vi "load system configuration.vi"(8 "error in":errorcluster) -> (0 "error out":errorcluster)   [LabVIEW 2015]
uses:
  global variables/params.vi
  <vilib>/Utility/config.llb/Read Key (String).vi
  <vilib>/Utility/config.llb/NI_LVConfig.lvlib
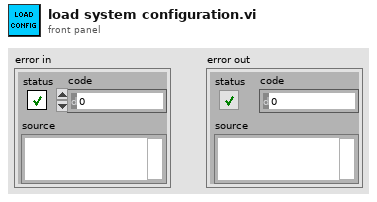
[diagram p1: front panel]
types:
  T1 = typedef "NI_LVConfig.lvlib/Config Data RefNum.ctl" = refnum<k1>
  T2 = cluster{"String":string, string, dbl, dbl, string, string, string, dbl, string}[]
  T3 = cluster{"String":string, string, dbl, dbl, string, string, string, dbl, string}
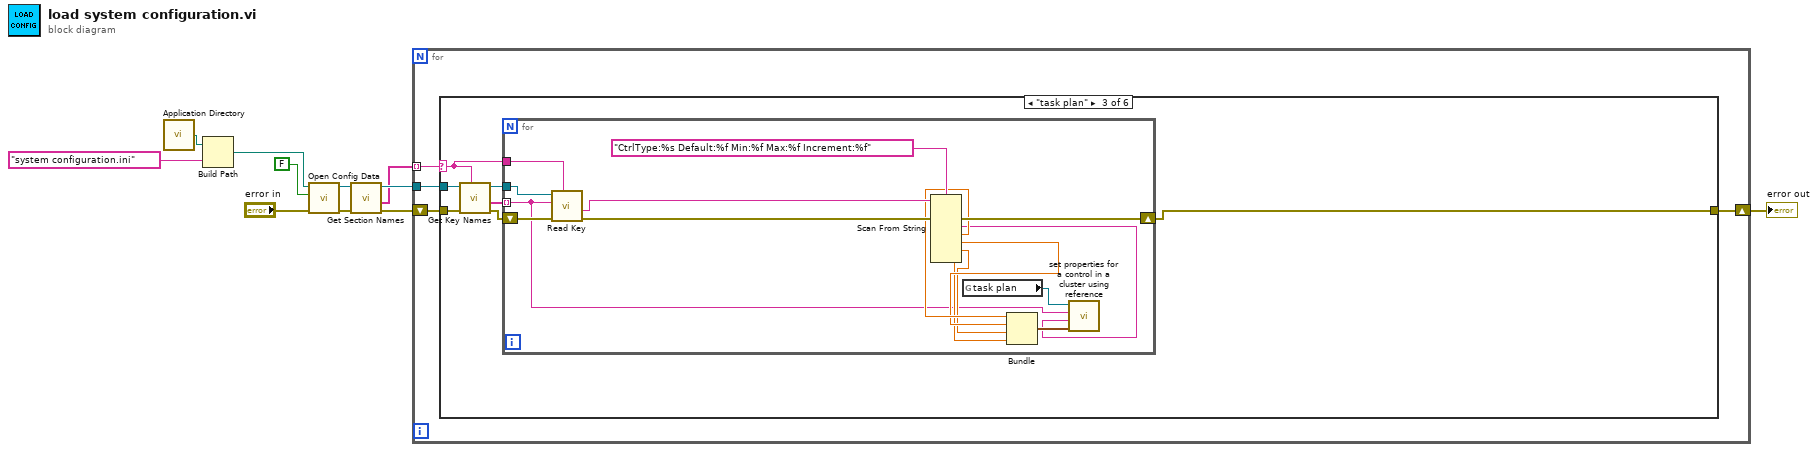
[diagram p0: block diagram]
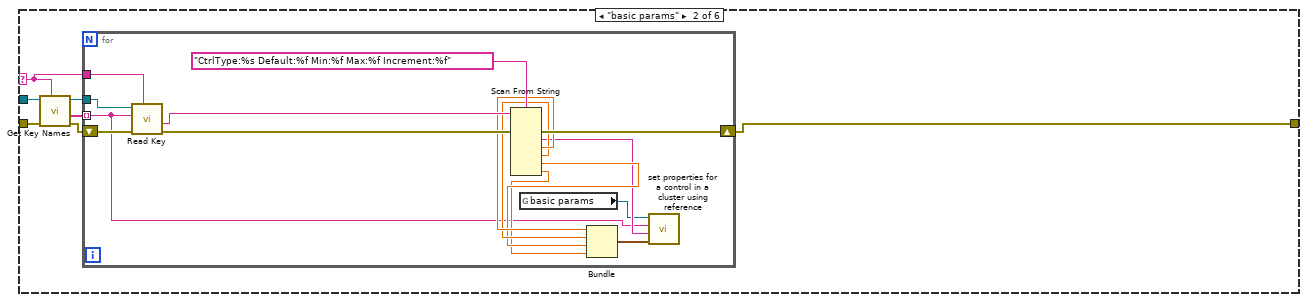
[diagram p3: hidden frame]
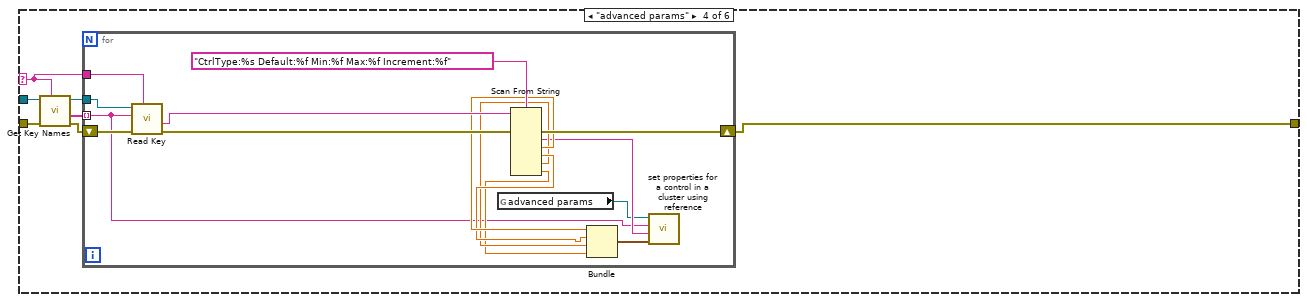
[diagram p4: hidden frame]
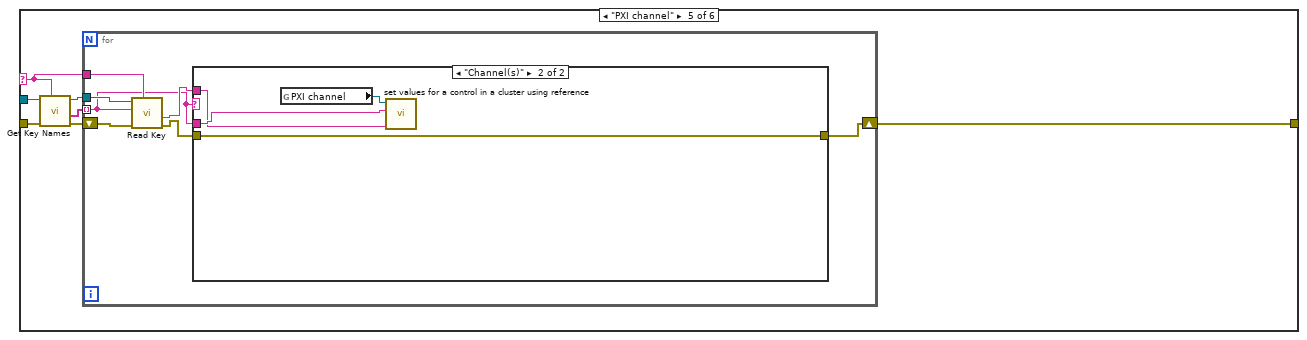
[diagram p5: hidden frame]
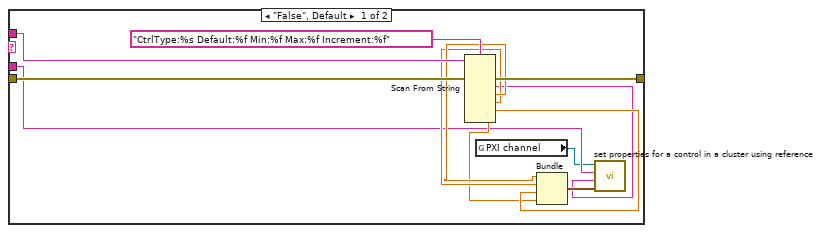
[diagram p6: hidden frame]
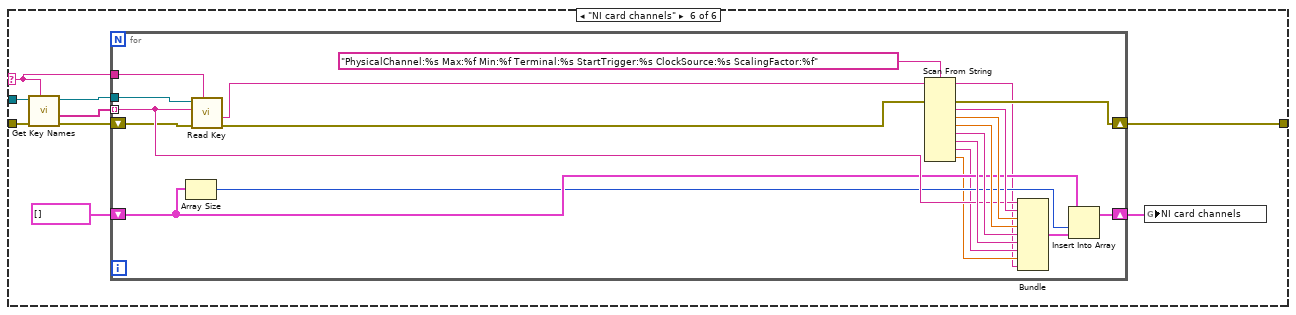
[diagram p7: hidden frame]
diagram:
  n1 = call <vilib>:"Application Directory.vi"() -> ("Application Directory"=w10:path)
  n2 = Build Path(base path=w10, name or relative path="system configuration.ini") -> (appended path=w8:path)
  n3 = call <vilib>:"Open Config Data.vi"("error in (no error)"="error in", "create file if necessary (T)"=FALSE, "configuration file path"=w8) -> ("error out"=w6:errorcluster, "refnum"=w5:T1)  [unwired: 6 in, 1 out]
  n4 = call <vilib>:"Get Section Names.vi"("error in (no error)"=w6, "refnum"=w5) -> ("error out"=w2:errorcluster, "section names"=w3:string[], "refnum out"=w4:T1)  [unwired: 7 in]
  n5 = for {
    tunnel: w3 -> [w15] mode=indexing
    tunnel: w4 -> [w14]
    shift-right: [w13] -> w1
    shift-left: w2 -> [w12]
    n6 = case shown="\"task plan\"" w15 {
      selector: w15 -> [_ w19 w41 w63 w85 w117]
      tunnel: w14 -> [_ w21 w43 w65 w87 w119]
      tunnel: w12 -> [w16 w20 w42 w64 w86 w118]
      tunnel: [w16 w17 w39 w61 w83 w115] -> w13
      frame "False", Default {
      }
      frame "basic params" {
        n7 = call <vilib>:"Get Key Names.vi"("section"=w19, "error in (no error)"=w20, "refnum"=w21) -> ("error out"=w18:errorcluster, "key names"=w23:string[], "refnum out"=w22:T1)  [unwired: 5 in, 1 out]
        n8 = for {
          tunnel: w23 -> [w25] mode=indexing
          tunnel: w22 -> [w38]
          tunnel: w19 -> [w34]
          shift-right: [w33] -> w17
          shift-left: w18 -> [w32]
          n9 = call-poly <vilib>:"Read Key.vi"("section"=w34, "error in (no error)"=w32, "key"=w25, "refnum"=w38) -> ("error out"=w36:errorcluster, "value"=w37:string)  [unwired: 4 in, 2 out]
          n10 = Scan From String(format string="CtrlType:%s Default:%f Min:%f Max:%f Increment:%f", input string=w37, error in=w36) -> (error out=w33:errorcluster, output 1=w26:string, output 2=w31:dbl, output 3=w30:dbl, output 4=w29:dbl, output 5=w28:dbl)  [unwired: 6 in, 2 out]
          n11 = global read "params.vi" "basic params"() -> (w24:refnum<vi>)
          n12 = Bundle(w31, w30, w29, w28) -> (w27:cluster{dbl, dbl, dbl, dbl})  [unwired: 1 in]
          n13 = call "set properties for a control in a cluster using reference.vi"("data entry"=w27, "type"=w26, "name"=w25, "Clust Refnum"=w24) -> ()  [unwired: 8 in]
        }
      }
      frame "task plan" {
        n14 = call <vilib>:"Get Key Names.vi"("section"=w41, "error in (no error)"=w42, "refnum"=w43) -> ("error out"=w40:errorcluster, "key names"=w45:string[], "refnum out"=w44:T1)  [unwired: 5 in, 1 out]
        n15 = for {
          tunnel: w45 -> [w47] mode=indexing
          tunnel: w44 -> [w60]
          tunnel: w41 -> [w56]
          shift-right: [w55] -> w39
          shift-left: w40 -> [w54]
          n16 = call-poly <vilib>:"Read Key.vi"("section"=w56, "error in (no error)"=w54, "key"=w47, "refnum"=w60) -> ("error out"=w58:errorcluster, "value"=w59:string)  [unwired: 4 in, 2 out]
          n17 = Scan From String(format string="CtrlType:%s Default:%f Min:%f Max:%f Increment:%f", input string=w59, error in=w58) -> (error out=w55:errorcluster, output 1=w48:string, output 2=w53:dbl, output 3=w52:dbl, output 4=w51:dbl, output 5=w50:dbl)  [unwired: 6 in, 2 out]
          n18 = global read "params.vi" "task plan"() -> (w46:refnum<vi>)
          n19 = Bundle(w53, w52, w51, w50) -> (w49:cluster{dbl, dbl, dbl, dbl})  [unwired: 1 in]
          n20 = call "set properties for a control in a cluster using reference.vi"("data entry"=w49, "type"=w48, "name"=w47, "Clust Refnum"=w46) -> ()  [unwired: 8 in]
        }
      }
      frame "advanced params" {
        n21 = call <vilib>:"Get Key Names.vi"("section"=w63, "error in (no error)"=w64, "refnum"=w65) -> ("error out"=w62:errorcluster, "key names"=w67:string[], "refnum out"=w66:T1)  [unwired: 5 in, 1 out]
        n22 = for {
          tunnel: w67 -> [w69] mode=indexing
          tunnel: w66 -> [w82]
          tunnel: w63 -> [w78]
          shift-right: [w77] -> w61
          shift-left: w62 -> [w76]
          n23 = call-poly <vilib>:"Read Key.vi"("section"=w78, "error in (no error)"=w76, "key"=w69, "refnum"=w82) -> ("error out"=w80:errorcluster, "value"=w81:string)  [unwired: 4 in, 2 out]
          n24 = global read "params.vi" "advanced params"() -> (w68:refnum<vi>)
          n25 = Scan From String(format string="CtrlType:%s Default:%f Min:%f Max:%f Increment:%f", input string=w81, error in=w80) -> (error out=w77:errorcluster, output 1=w70:string, output 2=w75:dbl, output 3=w74:dbl, output 4=w73:dbl, output 5=w72:dbl)  [unwired: 6 in, 2 out]
          n26 = Bundle(w75, w74, w73, w72) -> (w71:cluster{dbl, dbl, dbl, dbl})  [unwired: 1 in]
          n27 = call "set properties for a control in a cluster using reference.vi"("data entry"=w71, "type"=w70, "name"=w69, "Clust Refnum"=w68) -> ()  [unwired: 8 in]
        }
      }
      frame "PXI channel" {
        n28 = call <vilib>:"Get Key Names.vi"("section"=w85, "error in (no error)"=w86, "refnum"=w87) -> ("error out"=w84:errorcluster, "key names"=w89:string[], "refnum out"=w88:T1)  [unwired: 5 in, 1 out]
        n29 = for {
          tunnel: w89 -> [w90] mode=indexing
          tunnel: w88 -> [w96]
          tunnel: w85 -> [w93]
          shift-right: [w92] -> w83
          shift-left: w84 -> [w91]
          n30 = call-poly <vilib>:"Read Key.vi"("section"=w93, "error in (no error)"=w91, "key"=w90, "refnum"=w96) -> ("error out"=w94:errorcluster, "value"=w95:string)  [unwired: 4 in, 2 out]
          n31 = case shown="\"Channel(s)\"" w90 {
            tunnel: w95 -> [w108 w110]
            tunnel: w94 -> [w107 w109]
            tunnel: [w105 w109] -> w92
            tunnel: w90 -> [w98 w111]
            frame "False", Default {
              n32 = Scan From String(format string="CtrlType:%s Default:%f Min:%f Max:%f Increment:%f", input string=w108, error in=w107) -> (error out=w105:errorcluster, output 1=w99:string, output 2=w104:dbl, output 3=w103:dbl, output 4=w102:dbl, output 5=w101:dbl)  [unwired: 6 in, 2 out]
              n33 = global read "params.vi" "PXI channel"() -> (w97:refnum<vi>)
              n34 = Bundle(w104, w103, w102, w101) -> (w100:cluster{dbl, dbl, dbl, dbl})  [unwired: 1 in]
              n35 = call "set properties for a control in a cluster using reference.vi"("data entry"=w100, "type"=w99, "name"=w98, "Clust Refnum"=w97) -> ()  [unwired: 8 in]
            }
            frame "Channel(s)" {
              n36 = global read "params.vi" "PXI channel"() -> (w112:refnum<vi>)
              n37 = call "set values for a control in a cluster using reference.vi"("value"=w110, "name"=w111, "Clust Refnum"=w112) -> ()  [unwired: 9 in]
            }
          }
        }
      }
      frame "NI card channels" {
        n38 = call <vilib>:"Get Key Names.vi"("section"=w117, "error in (no error)"=w118, "refnum"=w119) -> ("error out"=w116:errorcluster, "key names"=w121:string[], "refnum out"=w120:T1)  [unwired: 5 in, 1 out]
        n39 = for {
          tunnel: w121 -> [w133] mode=indexing
          tunnel: w120 -> [w141]
          shift-right: [w132] -> w114
          shift-left: T2 [] -> [w131]
          tunnel: w117 -> [w128]
          shift-right: [w127] -> w115
          shift-left: w116 -> [w126]
          n40 = Array Size(array=w131) -> (size(s)=w130:i32)
          n41 = call-poly <vilib>:"Read Key.vi"("section"=w128, "error in (no error)"=w126, "key"=w133, "refnum"=w141) -> ("error out"=w139:errorcluster, "value"=w140:string)  [unwired: 4 in, 2 out]
          n42 = Scan From String(format string="PhysicalChannel:%s Max:%f Min:%f Terminal:%s StartTrigger:%s ClockSource:%s ScalingFactor:%f", input string=w140, error in=w139) -> (remaining string=w122:string, error out=w127:errorcluster, output 1=w138:string, output 2=w137:dbl, output 3=w136:dbl, output 4=w135:string, output 5=w134:string, output 6=w125:string, output 7=w123:dbl)  [unwired: 8 in, 1 out]
          n43 = Bundle("String"=w133, w138, w137, w136, w135, w134, w125, w123, w122) -> (w124:T3)  [unwired: 1 in]
          n44 = Insert Into Array(array=w131, index=w130, new element=w124) -> (w132:T2)
        }
        n45 = global write "params.vi" "NI card channels"(w114) -> ()
      }
    }
  }
  "error out" <- w1
